vi "Read SubComponent Data - Scaled.vi"(8 "error in (no error)":errorcluster, 11 "1553 SubComponent in":refnum<class "1553 SubComponent.lvclass">) -> (0 "error out":errorcluster, 1 "Scaled Data":dbl[](array[numeric]), 2 "Parameter":string[](array[string]), 3 "1553 SubComponent out":refnum<class "1553 SubComponent.lvclass">)   [LabVIEW 2020, in "BCI-1553 API.lvlib" / "1553 SubComponent.lvclass"]
doc: "This method returns the last data set read during the 'Retrieve SubComponent Data' and returns it as fully scaled double values as well as with a 1:1 parameter list the identifies what configuration parameter each data value is associated with."
uses:
  1553 SubComponent.lvclass
  1553 SubComponent.lvclass/1553 SubComponent.ctl
  Dependencies/Registry/Registry.lvclass/Registry.ctl
  Frames & Messages/TypeDefs/Parameter Table Data.ctl
  Frames & Messages/TypeDefs/Scaling Information.ctl
  BCI-1553 API.lvlib
  Dependencies/Registry/Registry.lvclass
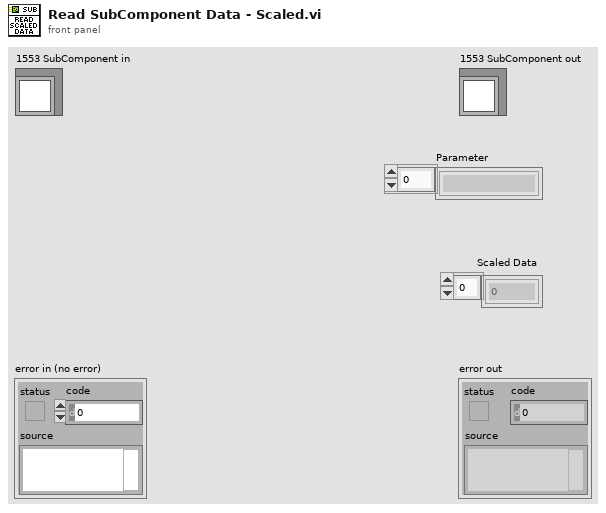
[diagram p1: front panel]
types:
  T1 = typedef "BCI-1553 API.lvlib/Parameter Table Data.ctl" = cluster{"Parameter Name":string, "Base Word":u16, "Address":u16, "Value":u64, "Mask":u16[], "Scaling Info":T2}
  T2 = typedef "BCI-1553 API.lvlib/Scaling Information.ctl" = cluster{"Bit Offset":i32, "Bit Count":i32, "LSB Resolution":dbl, "2's Complement":bool, "Big Endian":bool, "Sign Bit":bool}
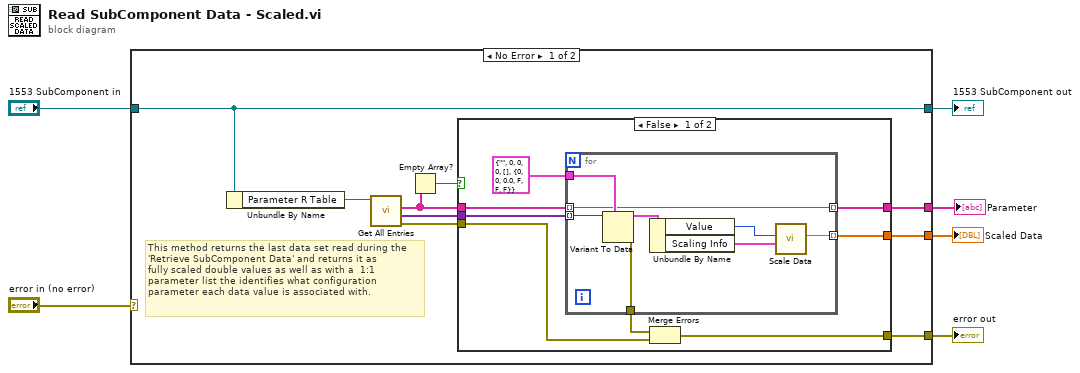
[diagram p0: block diagram]
diagram:
  n1 = case shown="No Error" "error in (no error)" {
    selector: "error in (no error)" -> [_ w34]
    tunnel: [w9 w34] -> w5
    tunnel: [w15 w33] -> w3
    tunnel: "1553 SubComponent in" -> [w15 w33]
    tunnel: [w12 _] -> w2
    tunnel: [w11 _] -> w1
    frame No Error {
      # "This method returns the last data set read during the\n'Retrieve SubComponent Data' and returns it as\nfully scaled double values as well as with a  1:1\nparameter list the identifies what configuration\nparameter each data value is associated with."
      n2 = Unbundle By Name(w15) -> ("Parameter R Table"=w13:refnum<class "Registry.lvclass">)
      n3 = call "Get All Entries.vi"("Registry in"=w13) -> ("error out"=w10:errorcluster, "Values"=w14:variant[], "Keys"=w8:string[])  [unwired: 8 in]
      n4 = Empty Array?(array=w8) -> (empty?=w7:bool)
      n5 = case shown="False" w7 {
        tunnel: w14 -> [w23 _]
        tunnel: [w21 _] -> w12
        tunnel: [w20 _] -> w11
        tunnel: w10 -> [w18 w32]
        tunnel: [w17 w32] -> w9
        tunnel: w8 -> [w16 _]
        frame False {
          n6 = for {
            tunnel: w16 -> [w26] mode=indexing
            tunnel: w23 -> [w31] mode=indexing
            tunnel: T1 {"Parameter Name"="", "Base Word"=0, "Address"=0, "Value"=0, "Mask"=[], "Scaling Info"={"Bit Offset"=0, "Bit Count"=0, "LSB Resolution"=0.0, "2's Complement"=FALSE, "Big Endian"=FALSE, "Sign Bit"=FALSE}} ("Parameter Table Data") -> [w30]
            tunnel: [w26] -> w20 mode=indexing
            tunnel: [w27] -> w21 mode=indexing
            tunnel: [w29] -> w19
            n7 = Variant To Data(type=w30, Variant=w31) -> (data=w24:T1, error out=w29:errorcluster)  [unwired: 1 in]
            n8 = Unbundle By Name(w24) -> ("Value"=w25:u64, "Scaling Info"=w28:T2)
            n9 = call "Scale Data.vi"("Scaling Info"=w28, "Raw Value"=w25) -> ("Scaled Value"=w27:dbl)  [unwired: 8 in, 1 out]
          }
          n10 = Merge Errors(w19, w18) -> (w17:errorcluster)
        }
        frame True {
          # "No op if there are no parameters."
        }
      }
    }
    frame Error {
    }
  }
  "error out" <- w5
  "1553 SubComponent out" <- w3
  "Scaled Data" <- w2
  "Parameter" <- w1
